vi "Usei.vi"() -> (0 "Boolean 4":bool, 1 "Boolean 3":bool, 2 "Boolean 2":bool, 3 "Boolean":bool)   [LabVIEW 2014]
uses:
  wlmData.dll
panel:
  out "Boolean 8":bool
  out "Boolean 7":bool
  out "Boolean 6":bool
  out "Boolean 5":bool
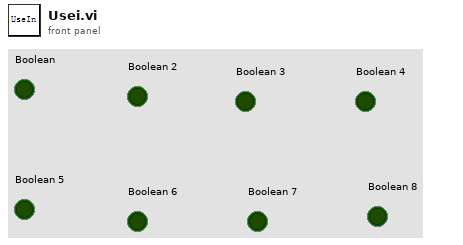
[diagram p1: front panel]
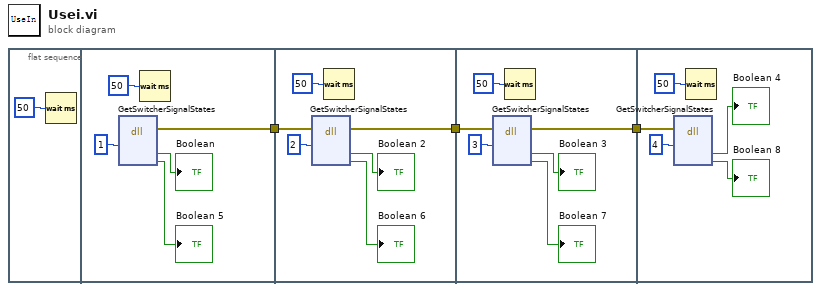
[diagram p0: block diagram]
diagram:
  n1 = flat-sequence {
    tunnel: [w5] -> w3
    tunnel: w3 -> [w11]
    tunnel: [w10] -> w2
    tunnel: w2 -> [w17]
    tunnel: [w16] -> w1
    tunnel: w1 -> [w22]
    frame #0 {
      n2 = Wait (ms)(milliseconds to wait=50) -> ()  [unwired: 1 out]
    }
    frame #1 {
      n3 = dll-call lib="wlmData.dll" fn="GetSwitcherSignalStates"("Siganal"=1) -> (error out=w5:errorcluster, "Boolean"=→"Boolean":bool, "Boolean 5"=→"Boolean 5":bool)  [unwired: 7 in, 1 out]
      n4 = Wait (ms)(milliseconds to wait=50) -> ()  [unwired: 1 out]
    }
    frame #2 {
      n5 = dll-call lib="wlmData.dll" fn="GetSwitcherSignalStates"(error in=w11, "Siganal"=2) -> (error out=w10:errorcluster, "Boolean 2"=→"Boolean 2":bool, "Boolean 6"=→"Boolean 6":bool)  [unwired: 6 in, 1 out]
      n6 = Wait (ms)(milliseconds to wait=50) -> ()  [unwired: 1 out]
    }
    frame #3 {
      n7 = dll-call lib="wlmData.dll" fn="GetSwitcherSignalStates"(error in=w17, "Siganal"=3) -> (error out=w16:errorcluster, "Boolean 3"=→"Boolean 3":bool, "Boolean 7"=→"Boolean 7":bool)  [unwired: 6 in, 1 out]
      n8 = Wait (ms)(milliseconds to wait=50) -> ()  [unwired: 1 out]
    }
    frame #4 {
      n9 = dll-call lib="wlmData.dll" fn="GetSwitcherSignalStates"(error in=w22, "Siganal"=4) -> ("Boolean 4"=→"Boolean 4":bool, "Boolean 8"=→"Boolean 8":bool)  [unwired: 6 in, 2 out]
      n10 = Wait (ms)(milliseconds to wait=50) -> ()  [unwired: 1 out]
    }
  }
